vi "Corr Digitizer to Meas Header.vi"(8 "error in":errorcluster, 11 "digitizer in":T1) -> (0 "error out":errorcluster, 2 "info data out":string, 3 "digitizer out":T1)   [LabVIEW 2013]
doc: "This VI will copy digitizer corrections to the measurement INFO header."
uses:
  Corr Digitizers.ctl
  octave/infolib.lvlibp/Private/Add key polymorph parts/String.vi
  octave/infolib.lvlibp
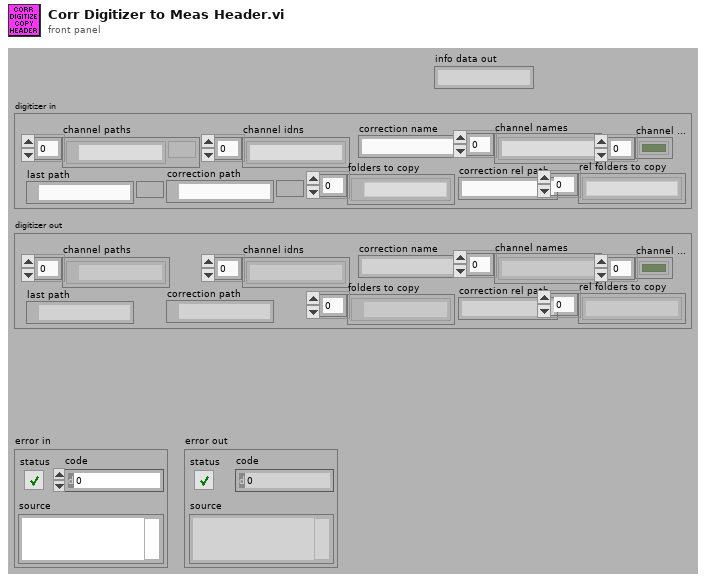
[diagram p1: front panel]
types:
  T1 = typedef "Corr Digitizers.ctl" = cluster{"last path":path, "channel paths":path[], "channel idns":string[], "correction name":string, "channel names":string[], "folders to copy":path[], "channel valid":bool[], "correction path":path, "correction rel path":string, "rel folders to copy":string[]}
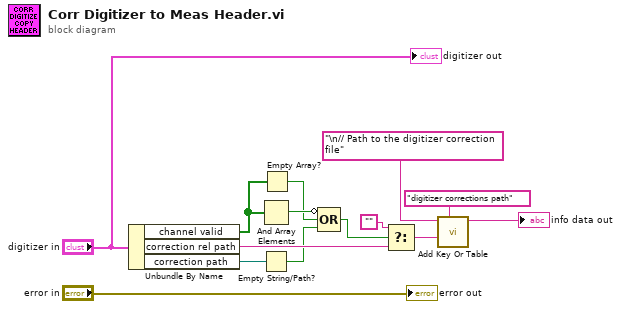
[diagram p0: block diagram]
diagram:
  n1 = Unbundle By Name("digitizer in") -> ("channel valid"=w3:bool[], "correction rel path"=w9:string, "correction path"=w10:path)
  n2 = And Array Elements(Boolean array=w3) -> (logical AND=w5:bool)
  n3 = Empty String/Path?(string/path=w10) -> (empty?=w4:bool)
  n4 = Empty Array?(array=w3) -> (empty?=w2:bool)
  n5 = Compound Arithmetic op=OR(invert w5, w2, w4) -> (w6:bool)
  n6 = Select(t="", s=w6, f=w9) -> (s? t:f=w7:string)
  n7 = call-poly "Add Key Or Table.vi"("key description"="digitizer corrections path", "string"=w7, "info data"="\n// Path to the digitizer correction file") -> ("info data out"=→"info data out":string)  [unwired: 7 in, 1 out]
  "error out" <- "error in"
  "digitizer out" <- "digitizer in"
